vi "CloseXL_Workbook.vi"(6 "Save? (F)":bool, 8 "error in (no error)":errorcluster, 10 "path":path, 11 "Refnum Cluster In":T1) -> (0 "error out":errorcluster, 3 "Refnum Cluster Out":T2)   [LabVIEW 2015]
doc: "This VI closes the XL worksheet previously opened by OpenXL_Worksheet.vi."
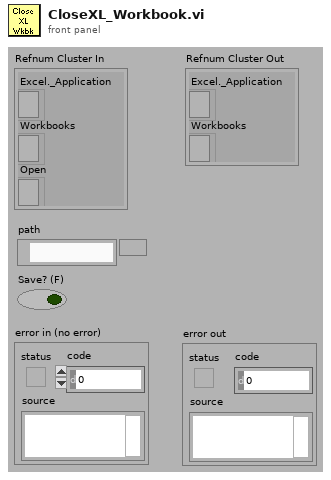
[diagram p1: front panel]
types:
  T1 = cluster{"Excel._Application":refnum<k7>, "Workbooks":refnum<k7>, "Open":refnum<k7>}
  T2 = cluster{"Excel._Application":refnum<k7>, "Workbooks":refnum<k7>}
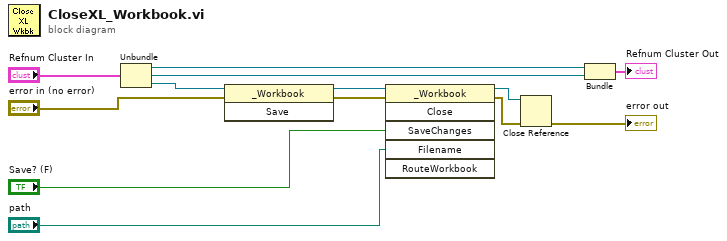
[diagram p0: block diagram]
diagram:
  n1 = Unbundle("Refnum Cluster In") -> ("Excel._Application"=w12:refnum<k7>, "Workbooks"=w11:refnum<k7>, "Open"=w10:refnum<k7>)
  n2 = invoke class="_Workbook" method="Save"(reference=w10, error in="error in (no error)") -> (reference out=w6:refnum<k7>, error out=w5:errorcluster)  [unwired: 1 in, 1 out]
  n3 = invoke class="_Workbook" method="Close"(reference=w6, error in=w5, "SaveChanges"="Save? (F)", "Filename"="path") -> (reference out=w2:refnum<k7>, error out=w1:errorcluster)  [unwired: 2 in, 4 out]
  n4 = Close Reference(reference=w2, error in (no error)=w1) -> (error out=→"error out":errorcluster)
  n5 = Bundle("Excel._Application"=w12, "Workbooks"=w11) -> (→"Refnum Cluster Out":T2)  [unwired: 1 in]
